vi "Initialize Reference Range Cart.vi"(8 "error in (no error)":errorcluster, 10 "Reference Range COM Port":refnum<visa-resource-name>, 11 "Reference Range Actor in":refnum<class "Reference Range Actor.lvclass">) -> (0 "error out":errorcluster, 3 "Reference Range Actor out":refnum<class "Reference Range Actor.lvclass">)   [LabVIEW 2018, in "Reference Range.lvlib" / "Reference Range Actor.lvclass"]
doc: "This VI is designed to initialize and open the COM Port that the motor controller is connected to. The default output value is Idle '128'."
uses:
  Reference Range Actor.lvclass
  C:/Program Files (x86)/National Instruments/LabVIEW 2018/vi.lib/ActorFramework/Actor/Actor.lvclass
  Reference Range Actor.lvclass/Reference Range Actor.ctl
  <vilib>/ActorFramework/Actor/Actor.lvclass/Actor.ctl
  <vilib>/Instr/_visa.llb/VISA Configure Serial Port (Instr).vi
  Range Controller Actor Messages/Send Log Message to Caller Msg/Send Log Message to Caller Msg.lvclass
  <vilib>/ActorFramework/Actor/Actor.lvclass
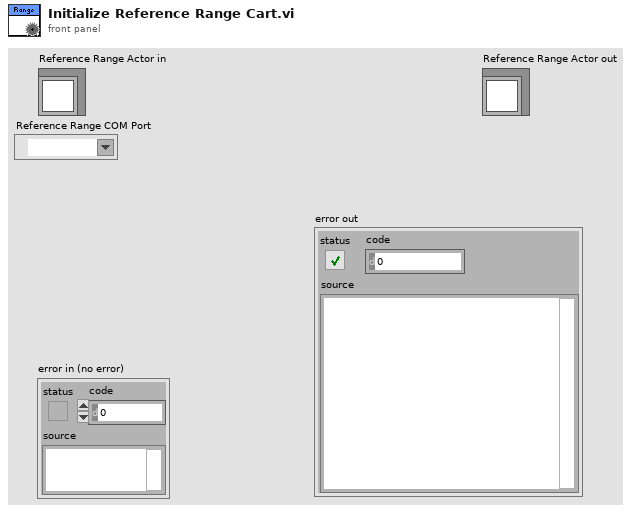
[diagram p1: front panel]
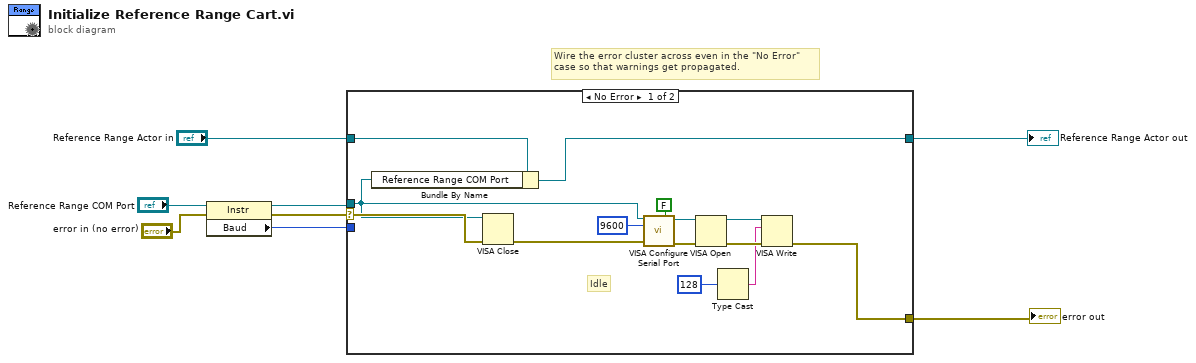
[diagram p0: block diagram]
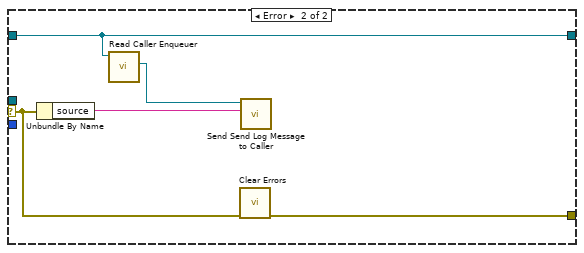
[diagram p2: hidden frame]
diagram:
  # "Wire the error cluster across even in the \"No Error\"\ncase so that warnings get propagated."
  n1 = property class="Instr"(reference="Reference Range COM Port", error in="error in (no error)") -> (reference out=w1:refnum<visa-resource-name>, error out=w3:errorcluster, "Baud"=w2:u32)
  n2 = case shown="No Error" w3 {
    selector: w3 -> [w12 w26]
    tunnel: [w17 w27] -> w6
    tunnel: [w9 w24] -> w7
    tunnel: "Reference Range Actor in" -> [w10 w24]
    tunnel: w1 -> [w11 _]
    tunnel: w2 -> [_ _]
    frame No Error {
      # "Idle"
      n3 = Bundle By Name(cluster=w10, "Reference Range COM Port"=w11) -> (w9:refnum<class "Reference Range Actor.lvclass">)
      n4 = VISA Close(VISA resource name=w11, error in (no error)=w12) -> (error out=w13:errorcluster)
      n5 = call-poly "VISA Configure Serial Port"("VISA resource name"=w11, "Enable Termination\nChar (T)"=FALSE ("Enable Termination\nChar (T)"), "baud rate (9600)"=u32 9600, "error in (no error)"=w13) -> ("VISA resource name out"=w19:refnum<visa-resource-name>, "error out"=w20:errorcluster)  [unwired: 10 in]
      n6 = VISA Open(error in (no error)=w20, VISA resource name=w19) -> (VISA resource name=w16:refnum<visa-resource-name>, error out=w18:errorcluster)  [unwired: 3 in]
      n7 = Type Cast(x=i16 128 ("Output State")) -> (*(type *) &x=w15:string)  [unwired: 1 in]
      n8 = VISA Write(VISA resource name=w16, write buffer=w15, error in (no error)=w18) -> (error out=w17:errorcluster)  [unwired: 2 out]
    }
    frame Error {
      n9 = Unbundle By Name(w26) -> ("source"=w23:string)
      n10 = call <vilib>:"Read Caller Enqueuer.vi"("Actor"=w24) -> ("Caller Enqueuer"=w25:refnum<class "Message Enqueuer.lvclass">)  [unwired: 10 in]
      n11 = call <vilib>:"Clear Errors.vi"("error in (no error)"=w26) -> ("error out"=w27:errorcluster)  [unwired: 5 in, 1 out]
      n12 = call "Send Send Log Message to Caller.vi"("Log Message"=w23, "Message Enqueuer in"=w25) -> ()  [unwired: 8 in, 2 out]
    }
  }
  "Reference Range Actor out" <- w7
  "error out" <- w6
